vi "Load.vi"(8 "error in (no error)":errorcluster, 11 "Config Name":string) -> (0 "error out":errorcluster)   [LabVIEW 2015, in "System Config.lvclass"]
uses:
  System Config.lvclass
  <vilib>/Utility/config.llb/NI_LVConfig.lvlib
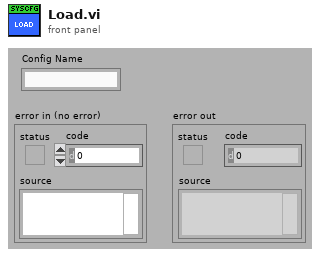
[diagram p1: front panel]
types:
  T1 = typedef "System Config.lvclass/ClassAttributesRef.ctl" = refnum<data-value>
  T2 = typedef "System Config.lvclass/ClassAttributes.ctl" = cluster{"Config":cluster{"Logging":cluster{"Log Files Directory":path, "Max Lines Per Log File":i32}, "Settings":T3}, "Core":cluster{"Config Directory":path, "Name":string, "Config Changed":refnum<user-event>}}
  T3 = typedef "System Config.lvclass/Settings.ctl" = cluster{"Dummy":dbl}
  T4 = cluster{"Logging":cluster{"Log Files Directory":path, "Max Lines Per Log File":i32}, "Settings":T3}
  T5 = typedef "NI_LVConfig.lvlib/Config Data RefNum.ctl" = refnum<k1>
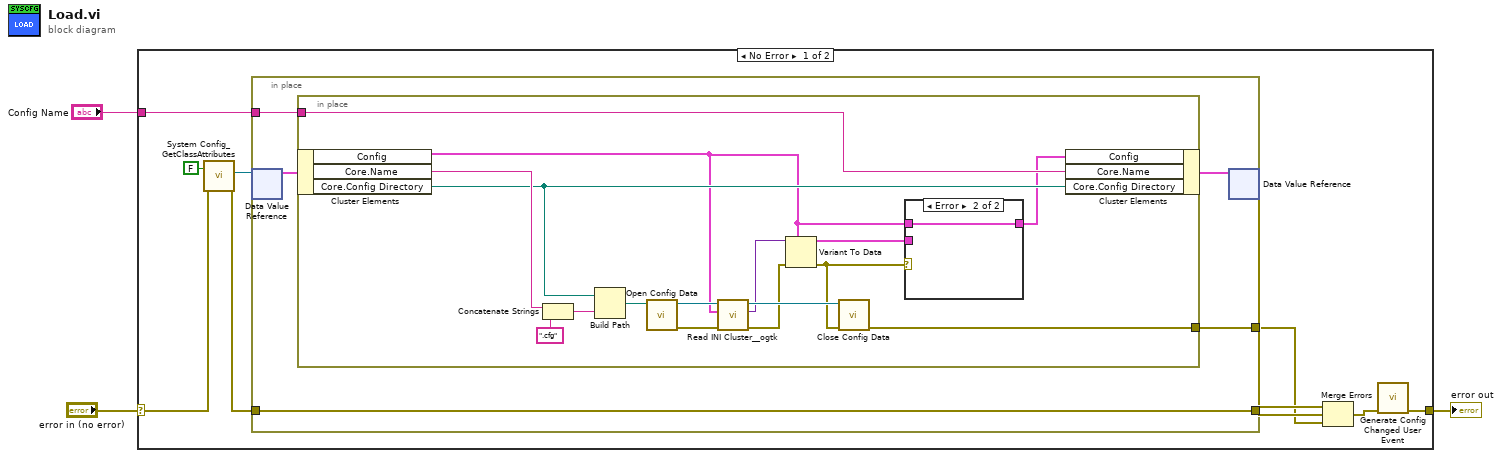
[diagram p0: block diagram]
diagram:
  n1 = case shown="No Error" "error in (no error)" {
    selector: "error in (no error)" -> [w13 w37]
    tunnel: [w5 w37] -> w2
    tunnel: "Config Name" -> [w7 _]
    frame No Error {
      n2 = call "System Config_GetClassAttributes.vi"("error in (no error)"=w13, "return data? (T)"=FALSE ("return data")) -> ("error out"=w12:errorcluster, "class attributes ref"=w11:T1)  [unwired: 6 in, 2 out]
      n3 = in-place {
        in-place-border: w12 -> [w16]
        in-place-border: [w16] -> w9
        in-place-border: w7 -> [w15]
        in-place-border: [w14] -> w4
        n4 = in-place-dvr #1(w11) -> (w17:T2)  [unwired: 1 out]
        n5 = in-place {
          in-place-border: w15 -> [w34]
          in-place-border: [w25] -> w14
          n6 = in-place-cluster #2(w17) -> ("Config"=w21:T4, "Core.Name"=w33:string, "Core.Config Directory"=w24:path)
          n7 = Concatenate Strings(w33, ".cfg" ("string")) -> (w31:string)
          n8 = Build Path(base path=w24, name or relative path=w31) -> (appended path=w30:path)
          n9 = call <vilib>:"Open Config Data.vi"("configuration file path"=w30) -> ("error out"=w27:errorcluster, "refnum"=w29:T5)  [unwired: 8 in, 1 out]
          n10 = call <userlib>:"Read INI Cluster__ogtk.vi"("error in (no error)"=w27, "INI Fomatted Cluster Type"=w21, "refnum"=w29) -> ("error out"=w20:errorcluster, "INI Fomatted Cluster"=w26:variant, "dup refnum"=w28:T5)  [unwired: 4 in, 2 out]
          n11 = Variant To Data(error in=w20, type=w21, Variant=w26) -> (data=w23:T4, error out=w19:errorcluster)
          n12 = call <vilib>:"Close Config Data.vi"("error in (no error)"=w19, "refnum"=w28) -> ("error out"=w25:errorcluster)  [unwired: 8 in, 1 out]
          n13 = case shown="Error" w19 {
            tunnel: w23 -> [w35 _]
            tunnel: [w35 w36] -> w22
            tunnel: w21 -> [_ w36]
            frame No Error {
            }
            frame Error {
            }
          }
          n14 = in-place-cluster #2("Config"=w22, "Core.Name"=w34, "Core.Config Directory"=w24) -> (w18:T2)
        }
        n15 = in-place-dvr #1(w18) -> (w8:errorcluster)  [unwired: 1 out]
      }
      n16 = Merge Errors(w9, w8, w4) -> (w6:errorcluster)
      n17 = call "Generate Config Changed User Event.vi"("error in (no error)"=w6) -> ("error out"=w5:errorcluster)  [unwired: 10 in]
    }
    frame Error {
    }
  }
  "error out" <- w2
